vi "Get Heading.vi"(7 "I2C Channel":u8, 8 "error in (no error)":errorcluster, 10 "Measurement Mode":enum16{"Standby Mode", "Continuous Mode"}(ring)=enum."Continuous Mode", 11 "LINX Resource In":T1) -> (0 "error out":errorcluster, 2 "Heading (deg)":dbl, 3 "LINX Resource Out":T1)   [LabVIEW 2014, in "LMH-LINX.lvlib" / "HMC6352.lvlib"]
uses:
  <vilib>/MakerHub/LINX/Public/Sensors/Orientation/Compass/HMC6352/HMC6352.lvlib
  <vilib>/MakerHub/LINX/Private/Type Defs/LINX Ref.ctl
  <vilib>/MakerHub/LINX/Private/Type Defs/Platform.ctl
  <vilib>/MakerHub/LINX/Private/Type Defs/Interface.ctl
  <vilib>/MakerHub/LINX/Private/Device/Type Defs/LINX Device Config.ctl
  <vilib>/MakerHub/LINX/Private/Device/Type Defs/TCP Config.ctl
  <vilib>/MakerHub/LINX/Private/Device/Type Defs/Channels.ctl
  <vilib>/MakerHub/LINX/Private/Local IO/LinxI2cWrite.vi
  <vilib>/MakerHub/LINX/Public/Utilities/Check Channel.vi
  <vilib>/MakerHub/LINX/Private/Utilties/Generate Error.vi
  <vilib>/MakerHub/LINX/LMH-LINX.lvlib
  <vilib>/MakerHub/LINX/Private/Device/Device.lvlib
panel:
  # "OUTPUTS"
  # "INPUTS"
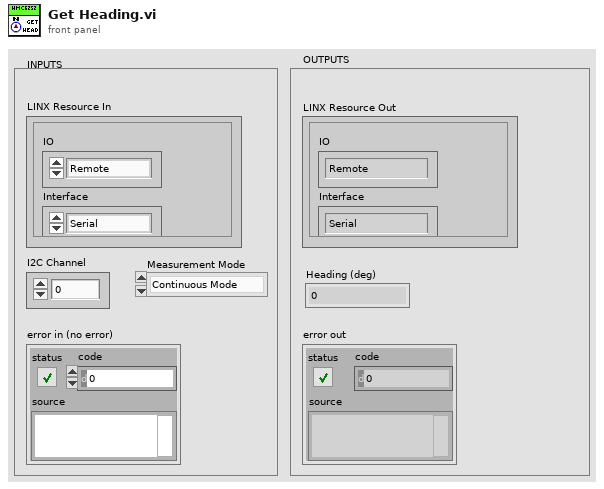
[diagram p1: front panel]
types:
  T1 = typedef "LMH-LINX.lvlib/LINX Ref.ctl" = cluster{"IO":T2, "Interface":T3, "LINX Device Config":T4}
  T2 = typedef "LMH-LINX.lvlib/Platform.ctl" = enum16{"Remote", "Local"}
  T3 = typedef "LMH-LINX.lvlib/Interface.ctl" = enum16{"Serial", "TCP"}
  T4 = typedef "LMH-LINX.lvlib/Device.lvlib/LINX Device Config.ctl" = cluster{"Interface":T3, "COM Port":refnum<visa-resource-name>, "TCP Configuration":T5, "Device Family":u8, "Device ID":u8, "Device Name":string, "TCP Ref":refnum<k5>, "Channels":T6}
  T5 = typedef "LMH-LINX.lvlib/Device.lvlib/TCP Config.ctl" = cluster{"IP Address":string, "Port":u16}
  T6 = typedef "LMH-LINX.lvlib/Channels.ctl" = cluster{"DI":u8[], "DO":u8[], "AI":u8[], "AO":u8[], "PWM":u8[], "QE":u8[], "UART":u8[], "I2C 2":u8[], "SPI":u8[], "CAN":u8[], "Servo":u8[], "AI Ref (V)":dbl, "AI Resolution (Bits)":u8, "AO Ref (V)":dbl, "AO Resolution (Bits)":u8}
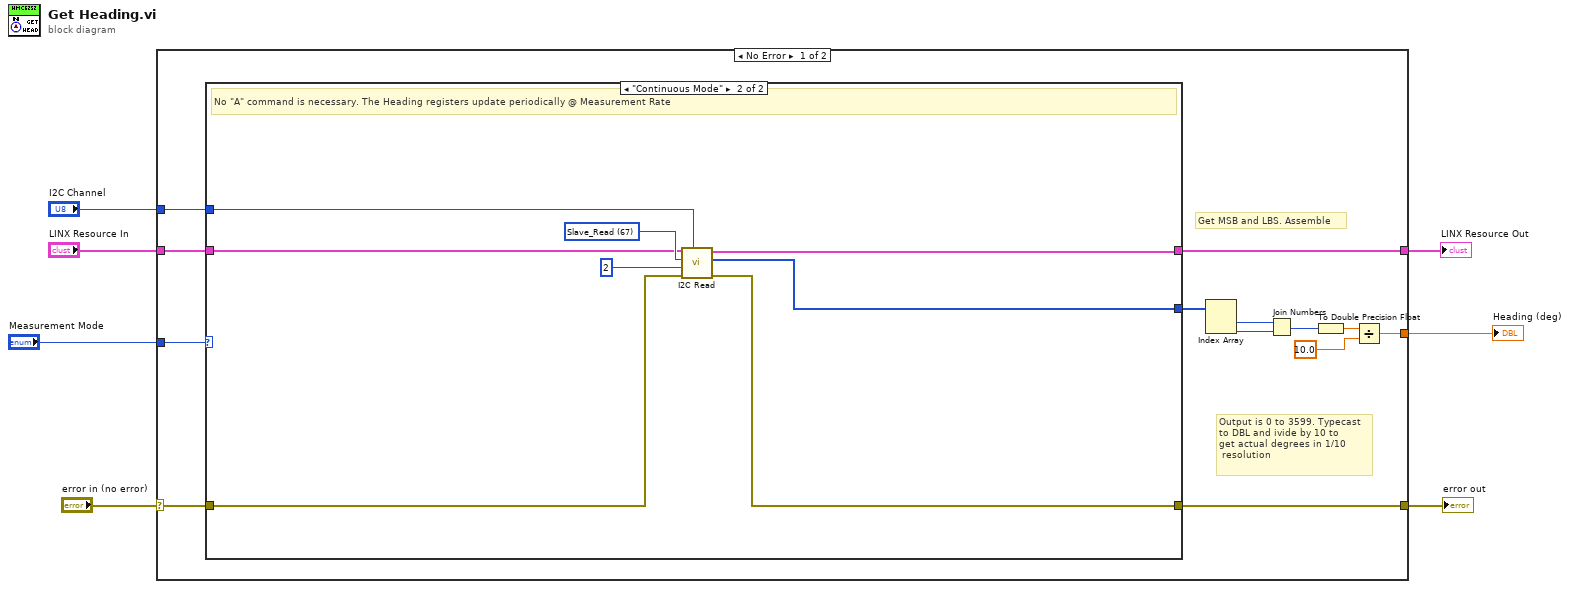
[diagram p0: block diagram]
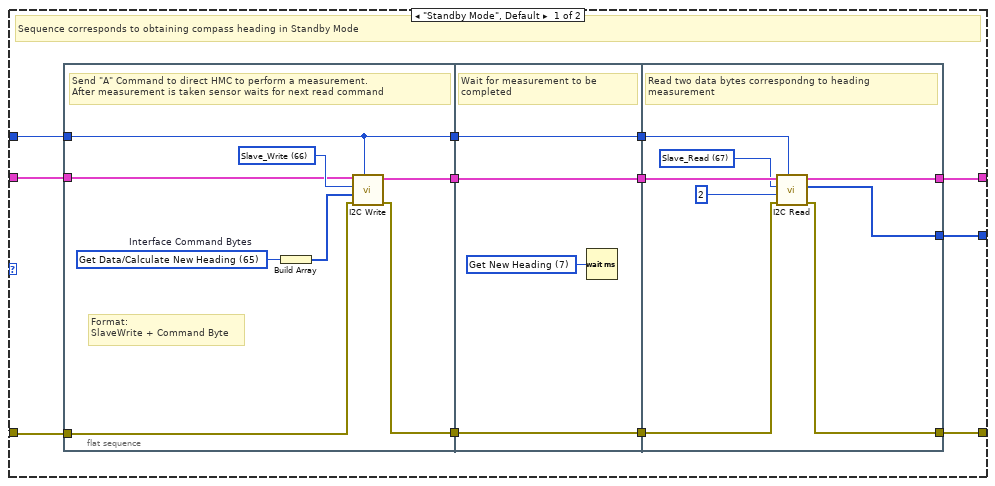
[diagram p2: hidden frame]
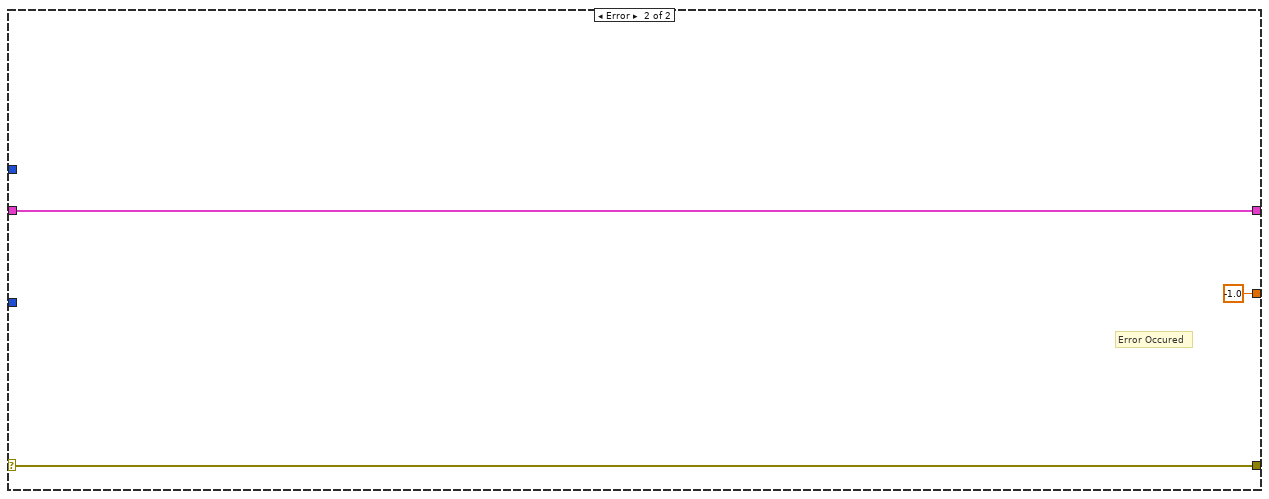
[diagram p3: hidden frame]
diagram:
  n1 = case shown="No Error" "error in (no error)" {
    selector: "error in (no error)" -> [w18 w63]
    tunnel: [w16 w63] -> w6
    tunnel: "LINX Resource In" -> [w20 w62]
    tunnel: "I2C Channel" -> [w19 _]
    tunnel: [w17 w62] -> w3
    tunnel: "Measurement Mode" -> [w15 _]
    tunnel: [w8 -1.0] -> w1
    frame No Error {
      # "Output is 0 to 3599. Typecast\nto DBL and ivide by 10 to\nget actual degrees in 1/10\n resolution"
      # "Get MSB and LBS. Assemble"
      n2 = case shown="\"Continuous Mode\"" w15 {
        tunnel: w20 -> [w31 w57]
        tunnel: w19 -> [w32 w58]
        tunnel: w18 -> [w30 w56]
        tunnel: [w29 w54] -> w17
        tunnel: [w28 w55] -> w16
        tunnel: [w21 w53] -> w14
        frame "Standby Mode", Default {
          # "Sequence corresponds to obtaining compass heading in Standby Mode"
          n3 = flat-sequence {
            tunnel: w32 -> [w33]
            tunnel: w31 -> [w37]
            tunnel: w30 -> [w36]
            tunnel: [w35] -> w27
            tunnel: [w34] -> w26
            tunnel: [w33] -> w22
            tunnel: w27 -> [w44]
            tunnel: w26 -> [w43]
            tunnel: [w44] -> w25
            tunnel: [w43] -> w24
            tunnel: [w41] -> w23
            tunnel: w22 -> [w41]
            tunnel: [w49] -> w28
            tunnel: [w51] -> w29
            tunnel: w25 -> [w52]
            tunnel: w24 -> [w50]
            tunnel: w23 -> [w48]
            tunnel: [w45] -> w21
            frame #0 {
              w39 = u8 65 items=["Write to EEPROM"=119, "Read from EEPROM"=114, "Write to RAM Register"=71, "Read from RAM Register"=103, "Enter Sleep Mode"=83, "Exit Sleep Mode"=87, "Update Bridge Offsets (Set/Reset)"=79, "Enter User Calibration Mode"=67, "Exit User Calibration Mode"=69, "Save Operation Mode to EEPROM"=76, "Get Data/Calculate New Heading"=65]  # Interface Command Bytes
              w38 = u8 66 items=["Slave_Write"=66, "Slave_Read"=67] ("HMC6352 Slave Address")
              # "Format:\nSlaveWrite + Command Byte"
              # "Send \"A\" Command to direct HMC to perform a measurement.\nAfter measurement is taken sensor waits for next read command"
              n4 = Build Array(w39) -> (w40:u8[])
              n5 = call <vilib>:"I2C Write.vi"("I2C Channel"=w33, "Error In"=w36, "Data"=w40, "I2C Slave Address (0)"=w38, "LINX Resource"=w37) -> ("Error Out"=w34:errorcluster, "LINX Resource"=w35:T1)  [unwired: 5 in]
            }
            frame #1 {
              w42 = u32 7 items=["Update Bridge Offsets"=6, "Exit User Calibration Mode"=14, "Get New Heading"=7] ("Command Time Delays (ms)")
              # "Wait for measurement to be completed"
              n6 = Wait (ms)(milliseconds to wait=w42) -> ()  [unwired: 1 out]
            }
            frame #2 {
              w47 = u8 67 items=["Slave_Write"=66, "Slave_Read"=67] ("HMC6352 Slave Address")
              # "Read two data bytes correspondng to heading measurement"
              n7 = call <vilib>:"I2C Read.vi"("I2C Channel"=w48, "Error In"=w50, "Bytes To Read"=u8 2, "I2C Slave Address (0)"=w47, "LINX Resource"=w52) -> ("Error Out"=w49:errorcluster, "Data"=w45:u8[], "LINX Resource"=w51:T1)  [unwired: 4 in]
            }
          }
        }
        frame "Continuous Mode" {
          w60 = u8 67 items=["Slave_Write"=66, "Slave_Read"=67] ("HMC6352 Slave Address")
          # "No \"A\" command is necessary. The Heading registers update periodically @ Measurement Rate"
          n8 = call <vilib>:"I2C Read.vi"("I2C Channel"=w58, "Error In"=w56, "Bytes To Read"=u8 2, "I2C Slave Address (0)"=w60, "LINX Resource"=w57) -> ("Error Out"=w55:errorcluster, "Data"=w53:u8[], "LINX Resource"=w54:T1)  [unwired: 4 in]
        }
      }
      n9 = Index Array(array=w14) -> (element #1=w13:u8, element #2=w12:u8)  [unwired: 2 in]
      n10 = Join Numbers(hi=w13, lo=w12) -> ((hi.lo)=w11:u16)
      n11 = To Double Precision Float(number=w11) -> (double precision float=w10:dbl)
      n12 = Divide(x=w10, y=10.0) -> (x/y=w8:dbl)
    }
    frame Error {
      # "Error Occured"
    }
  }
  "error out" <- w6
  "LINX Resource Out" <- w3
  "Heading (deg)" <- w1
